vi "MathResizeProportional.vi"(8 "error in (no error)":errorcluster, 9 "Old PanelBounds":T2, 10 "New PanelBounds":T2) -> (0 "error out":errorcluster, 1 "Old dimensions":T1, 2 "New dimensions":T1, 4 "dHeight >= dWidth":bool, 5 "IncreasingPanel":bool)   [LabVIEW 2016]
uses:
  <vilib>/Utility/miscctls.llb/LVRectTypeDef.ctl
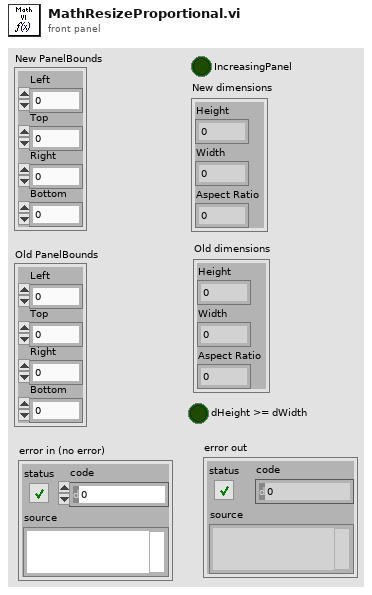
[diagram p1: front panel]
types:
  T1 = cluster{"Height":i16, "Width":i16, "Aspect Ratio":dbl}
  T2 = typedef "LVRectTypeDef.ctl" = cluster{"Left":i16, "Top":i16, "Right":i16, "Bottom":i16}
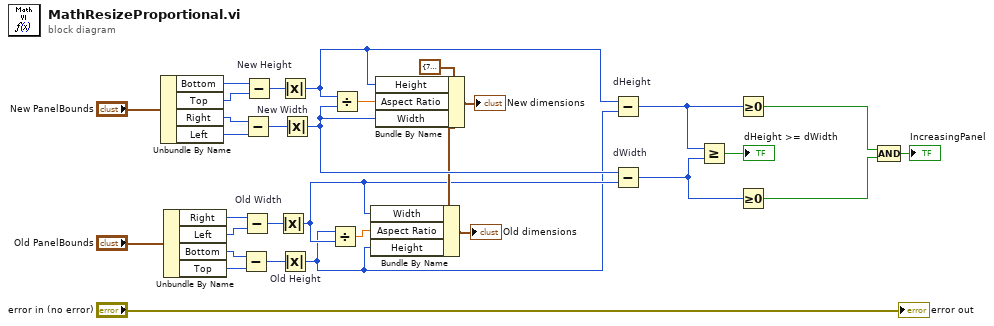
[diagram p0: block diagram]
diagram:
  w13 = T1 {"Height"=750, "Width"=500, "Aspect Ratio"=1.5} ("New dimensions")
  n1 = Unbundle By Name("New PanelBounds") -> ("Bottom"=w30:i16, "Top"=w29:i16, "Right"=w26:i16, "Left"=w27:i16)
  n2 = Unbundle By Name("Old PanelBounds") -> ("Right"=w22:i16, "Left"=w21:i16, "Bottom"=w20:i16, "Top"=w19:i16)
  n3 = Subtract(x=w20, y=w19) -> (x-y=w24:i16)
  n4 = Subtract(x=w22, y=w21) -> (x-y=w23:i16)
  n5 = Subtract(x=w26, y=w27) -> (x-y=w25:i16)
  n6 = Subtract(x=w30, y=w29) -> (x-y=w28:i16)
  n7 = Absolute Value "Old Width"(x=w23) -> (abs(x)=w11:i16)
  n8 = Absolute Value "New Height"(x=w28) -> (abs(x)=w16:i16)
  n9 = Absolute Value "Old Height"(x=w24) -> (abs(x)=w10:i16)
  n10 = Absolute Value "New Width"(x=w25) -> (abs(x)=w14:i16)
  n11 = Divide(x=w10, y=w11) -> (x/y=w12:dbl)
  n12 = Divide(x=w16, y=w14) -> (x/y=w15:dbl)
  n13 = Bundle By Name(cluster=w13, "Width"=w11, "Aspect Ratio"=w12, "Height"=w10) -> (→"Old dimensions":T1)
  n14 = Bundle By Name(cluster=w13, "Height"=w16, "Aspect Ratio"=w15, "Width"=w14) -> (→"New dimensions":T1)
  n15 = Subtract "dHeight"(x=w16, y=w10) -> (x-y=w6:i16)
  n16 = Subtract "dWidth"(x=w14, y=w11) -> (x-y=w5:i16)
  n17 = Greater Or Equal?(x=w6, y=w5) -> (x >= y?=→"dHeight >= dWidth":bool)
  n18 = Greater Or Equal To 0?(x=w6) -> (x >= 0?=w4:bool)
  n19 = Greater Or Equal To 0?(x=w5) -> (x >= 0?=w3:bool)
  n20 = Compound Arithmetic op=AND(w4, w3) -> (→"IncreasingPanel":bool)
  "error out" <- "error in (no error)"
